vi "Execution-handler.vi"(8 "error in (no error)":errorcluster, 11 "Object ref in":T1) -> (0 "error out":errorcluster, 3 "Object ref out":T1)   [LabVIEW 2013, in "PowderDeposition.lvlib" / "PD-Main.lvclass"]
uses:
  PD-Main.lvclass
  Object-reference.ctl
  Execution-actions.ctl
  Client-status.ctl
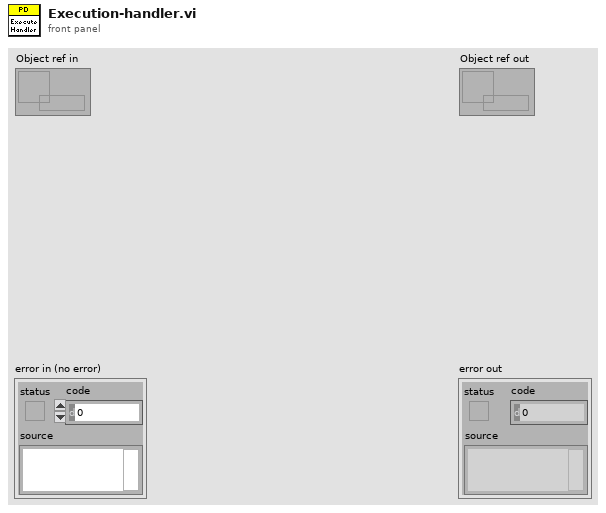
[diagram p1: front panel]
types:
  T1 = typedef "PowderDeposition.lvlib/PD-Main.lvclass/Object-reference.ctl" = refnum<data-value>
  T2 = typedef "PowderDeposition.lvlib/PD-Main.lvclass/Execution-actions.ctl" = enum16{"Idle", "Execute action", "Execute sequence", "Execute seq with assert", "Exit"}
  T3 = typedef "PowderDeposition.lvlib/PD-Main.lvclass/Client-status.ctl" = enum16{"Idle", "Initialized", "Configured", "Activated", "Started", "Paused", "Stopped", "Reset", "Error", "Exited"}
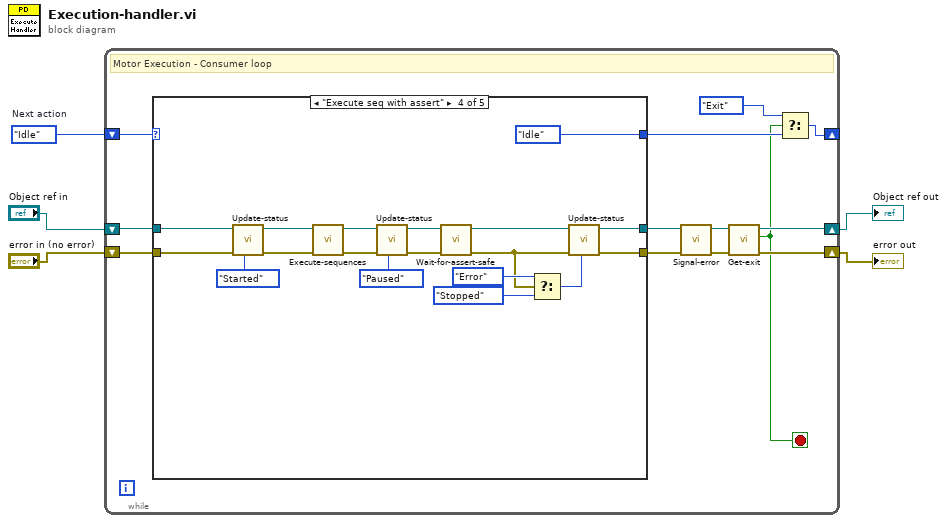
[diagram p0: block diagram]
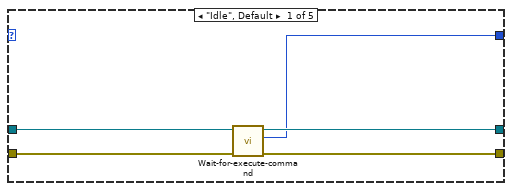
[diagram p2: hidden frame]
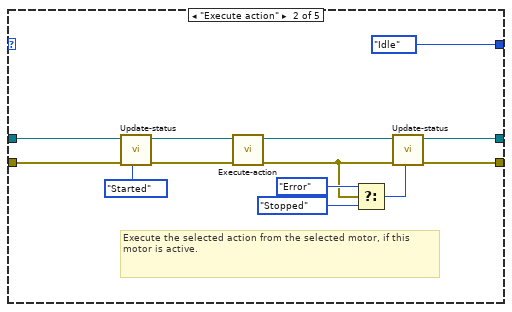
[diagram p3: hidden frame]
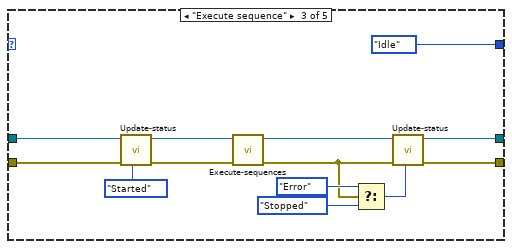
[diagram p4: hidden frame]
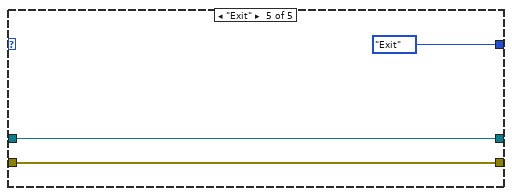
[diagram p5: hidden frame]
diagram:
  w5 = Execution-actions."Idle"  # Next action
  n1 = while {
    shift-right: [w10] -> _
    shift-left: w5 -> [w18]
    shift-right: [w8] -> w4
    shift-left: "error in (no error)" -> [w17]
    shift-right: [w13] -> w3
    shift-left: "Object ref in" -> [w16]
    stop <- w6 stop-if-true
    # "Motor Execution - Consumer loop"
    n2 = case shown="\"Execute seq with assert\"" w18 {
      tunnel: w17 -> [w19 w33 w43 w62 w68]
      tunnel: [w21 w24 w37 w57 w68] -> w7
      tunnel: [w20 Execution-actions."Idle" ("Action Handler states") Execution-actions."Idle" ("Action Handler states") Execution-actions."Idle" ("Action Handler states") Execution-actions."Exit" ("Action Handler states")] -> w11
      tunnel: w16 -> [w23 w34 w44 w65 w69]
      tunnel: [w22 w25 w39 w58 w69] -> w15
      frame "Idle", Default {
        n3 = call "Wait-for-execute-command.vi"("error in (no error)"=w19, "Object ref in"=w23) -> ("error out"=w21:errorcluster, "Next execution"=w20:T2, "Object ref out"=w22:T1)  [unwired: 7 in]
      }
      frame "Execute action" {
        # "Execute the selected action from the selected motor, if this motor is active."
        n4 = call "Update-status.vi"("Status"=Client-status."Started", "error in (no error)"=w33, "Object ref in"=w34) -> ("error out"=w32:errorcluster, "Object ref out"=w31:T1)  [unwired: 7 in]
        n5 = call "Execute-action.vi"("error in (no error)"=w32, "Object ref in"=w31) -> ("error out"=w27:errorcluster, "Object ref out"=w26:T1)  [unwired: 8 in]
        n6 = Select(t=Client-status."Error", s=w27, f=Client-status."Stopped" ("Status")) -> (s? t:f=w29:T3)
        n7 = call "Update-status.vi"("Status"=w29, "error in (no error)"=w27, "Object ref in"=w26) -> ("error out"=w24:errorcluster, "Object ref out"=w25:T1)  [unwired: 7 in]
      }
      frame "Execute sequence" {
        n8 = call "Update-status.vi"("Status"=Client-status."Started", "error in (no error)"=w43, "Object ref in"=w44) -> ("error out"=w42:errorcluster, "Object ref out"=w41:T1)  [unwired: 7 in]
        n9 = call "Execute-sequences.vi"("error in (no error)"=w42, "Object ref in"=w41) -> ("error out"=w38:errorcluster, "Object ref out"=w40:T1)  [unwired: 8 in]
        n10 = Select(t=Client-status."Error", s=w38, f=Client-status."Stopped" ("Status")) -> (s? t:f=w47:T3)
        n11 = call "Update-status.vi"("Status"=w47, "error in (no error)"=w38, "Object ref in"=w40) -> ("error out"=w37:errorcluster, "Object ref out"=w39:T1)  [unwired: 7 in]
      }
      frame "Execute seq with assert" {
        n12 = call "Update-status.vi"("Status"=Client-status."Started", "error in (no error)"=w62, "Object ref in"=w65) -> ("error out"=w63:errorcluster, "Object ref out"=w64:T1)  [unwired: 7 in]
        n13 = call "Execute-sequences.vi"("error in (no error)"=w63, "Object ref in"=w64) -> ("error out"=w52:errorcluster, "Object ref out"=w53:T1)  [unwired: 8 in]
        n14 = call "Update-status.vi"("Status"=Client-status."Paused", "error in (no error)"=w52, "Object ref in"=w53) -> ("error out"=w51:errorcluster, "Object ref out"=w50:T1)  [unwired: 7 in]
        n15 = call "Wait-for-assert-safe.vi"("error in (no error)"=w51, "Object ref in"=w50) -> ("error out"=w56:errorcluster, "Object ref out"=w55:T1)  [unwired: 8 in]
        n16 = Select(t=Client-status."Error", s=w56, f=Client-status."Stopped" ("Status")) -> (s? t:f=w60:T3)
        n17 = call "Update-status.vi"("Status"=w60, "error in (no error)"=w56, "Object ref in"=w55) -> ("error out"=w57:errorcluster, "Object ref out"=w58:T1)  [unwired: 7 in]
      }
      frame "Exit" {
      }
    }
    n18 = call "Signal-error.vi"("error in (no error)"=w7, "Data in"=w15) -> ("error out"=w12:errorcluster, "Data out"=w14:T1)  [unwired: 8 in]
    n19 = call "Get-exit.vi"("error in (no error)"=w12, "Object ref in"=w14) -> ("error out"=w8:errorcluster, "Exit?"=w6:bool, "Object ref out"=w13:T1)  [unwired: 7 in]
    n20 = Select(t=Execution-actions."Exit", s=w6, f=w11) -> (s? t:f=w10:T2)
  }
  "error out" <- w4
  "Object ref out" <- w3
